vi "Vision Processing Broken.vi"(4 "error in (no error)":errorcluster, 7 "Image Size":T1=enum."320x240") -> ()   [LabVIEW 2015]
doc: "This VI runs in parallel to other tasks. It gets images from the camera, processes them for color or shape and uses commands or globals to affect the behavior of other subsystems."
uses:
  <vilib>/Rock Robotics/WPI/Camera/WPI_CameraImageSize.ctl
  Vision Support Code/Camera Types.ctl
  <vilib>/Rock Robotics/WPI/Camera/WPI_CameraWhite Balance Values.ctl
  <vilib>/Rock Robotics/WPI/Camera/WPI_CameraExposure Values.ctl
  <vilib>/Rock Robotics/WPI/Camera/WPI_CameraFrameRate.ctl
  Framework/Robot Global Data.vi
  Drive/Implementation/Global Drive Variables.vi
  LED Lights/LED Lights Global.vi
  <vilib>/vision/NI_Vision_Development_Module.lvlib
panel:
  out "error out 2":errorcluster
  out "error out":errorcluster
  out "Vision Enabled":bool
  in  "Max Limit %":dbl=0.12 format="%#_13g"
  in  "Min Limit %":dbl=0.12 format="%#_13g"
  in  "Image Size 2":T1=enum."320x240"
  out "ms to process 2":u32
  in  "error in (no error) 2":errorcluster
  out "ms to process":u32
  in  "LED Color":T2={"Hue"={23.67058792990901, 48.923317529462665}, "Sat"={66.78571428571429, 255.0}, "Val"={48.571428571428584, 255.0}} {"Hue" scale=0.0..255.0 scale format="%#_3g"}
  out "Qualified Particles":i32
  in  "Score Threshold":dbl=75.0
  in  "Aspect Fudge Factor":dbl=1.0
  in  "Min Score Threshold":i32=75
  in  "Camera Type":T3=enum."MS HD3000 square"
  in  "Emphasize Limit Tests":bool=TRUE
  out "Masked 2":T4(plugin-control)
  in  "Display Mask":bool=TRUE
  out "Original Image":T4(plugin-control)
  in  "Display Original":bool=TRUE
  out "Sorted Particle Scores":T5(array[cluster]) {"Moment Factor" format="%#_3g"; "Aspect Ratio" format="%#_3g"; "Area to CH" format="%#_3g"; "X" format="%#_3g"; "Y" format="%#_3g"}
  out "Highest Avg Score":dbl
  out "Detected Targets":T6(array[cluster]) {"Normalized Rect"."Numeric 5" format="%#_2g"; "Normalized Rect"."Numeric 3" format="%#_2g"; "Normalized Rect"."Numeric 2" format="%#_2g"; "Normalized Rect"."Numeric" format="%#_2g"}
  out "fps":dbl
  out "Masked":T4(plugin-control)
  # "Density Profile"
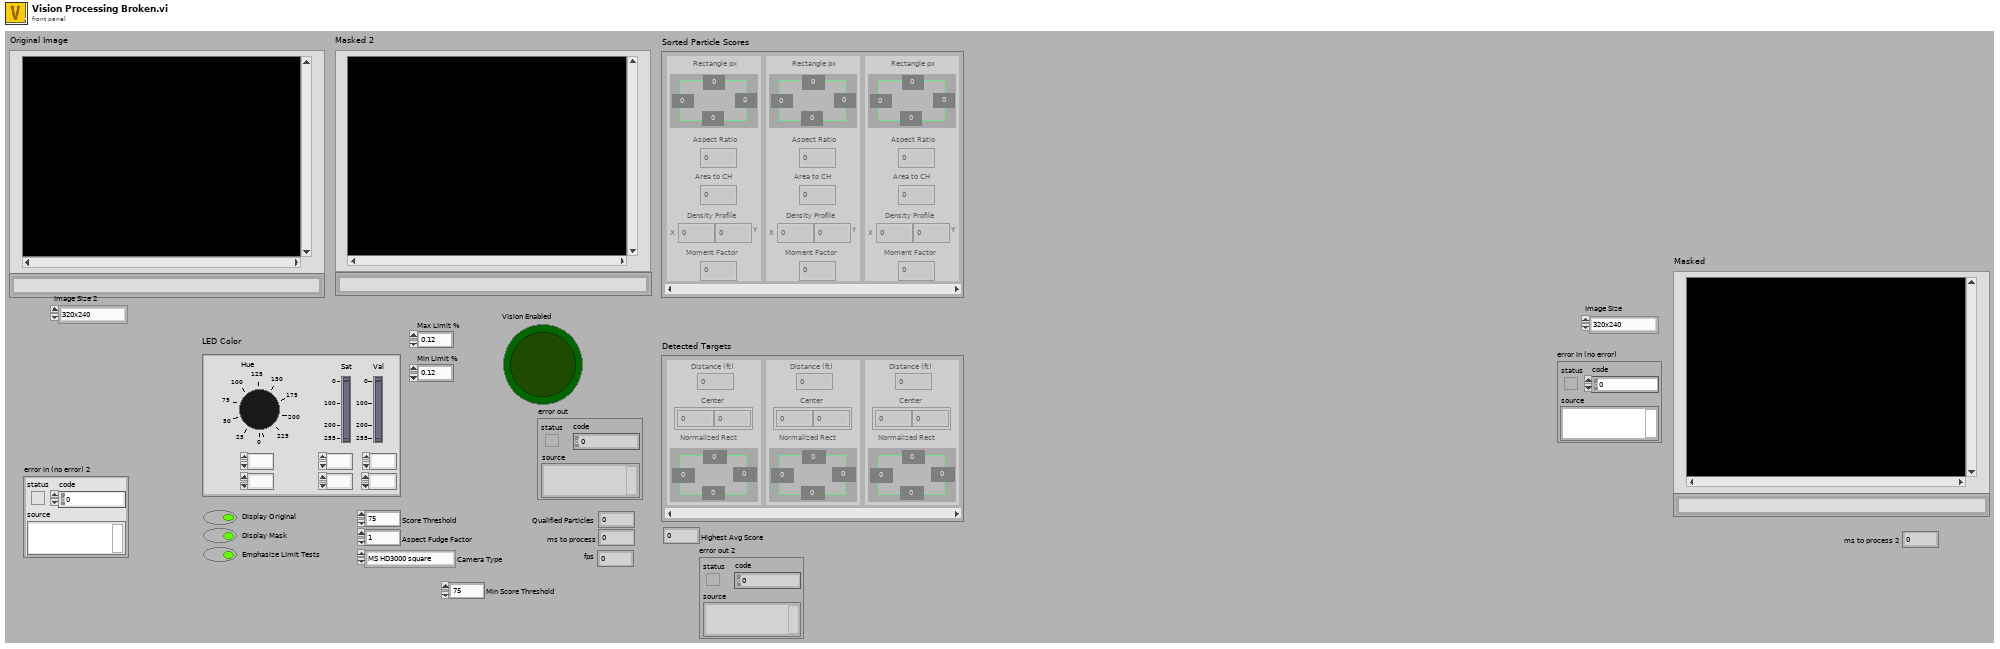
[diagram p1: front panel]
types:
  T1 = typedef "WPI_CameraImageSize.ctl" = enum16{"640x480", "320x240", "160x120", "Custom"}
  T2 = cluster{"Hue":cluster{dbl, dbl}, "Sat":cluster{dbl, dbl}, "Val":cluster{dbl, dbl}}
  T3 = typedef "Camera Types.ctl" = enum16{"206", "1011", "1013", "MS HD3000 square", "MS HD3000 640x480"}
  T4 = typedef "IMAQ Image.ctl" = refnum<image>
  T5 = cluster{"Rectangle px":cluster{"Numeric":dbl, "Numeric 2":dbl, "Numeric 3":dbl, "Numeric 5":dbl}, "Aspect Ratio":dbl, "Area to CH":dbl, "X":dbl, "Y":dbl, "Moment Factor":dbl}[]
  T6 = cluster{"Distance (ft)":dbl, "Center":cluster{dbl, dbl}, "Normalized Rect":cluster{"Numeric":dbl, "Numeric 2":dbl, "Numeric 3":dbl, "Numeric 5":dbl}}[]
  T7 = typedef "WPI_CameraFrameRate.ctl" = u32
  T8 = typedef "WPI_CameraExposure Values.ctl" = enum16{"Auto", "Flicker-free 50 Hz", "Flicker-free 60 Hz", "Hold current", "Custom"}
  T9 = typedef "WPI_CameraWhite Balance Values.ctl" = enum16{"Auto", "Fixed indoor", "Fixed outdoor 1", "Fixed outdoor 2", "Fixed fluorescent 1", "Fixed fluorescent 2", "Hold current", "Custom"}
  T10 = typedef "WPI_CameraDevRef.ctl" = cluster{"Camera Address":string, "CameraStatus":errorcluster}
  T11 = typedef "Image Type" = u32
  T12 = typedef "Particle Parameters" = i32
  T13 = cluster{"Bounding box":cluster{"left":dbl, "top":dbl, "right":dbl, "bottom":dbl}, "Aspect Ratio":dbl, "Area to CH":dbl, "X Mask":dbl, "Y Mask":dbl, "Moment":dbl}[]
  T14 = cluster{"Rectangle":cluster{"Numeric":dbl, "Numeric 2":dbl, "Numeric 3":dbl, "Numeric 5":dbl}, "L":dbl, "Area to CH":dbl, "X":dbl, "Y":dbl, "Moment Factor":dbl}[]
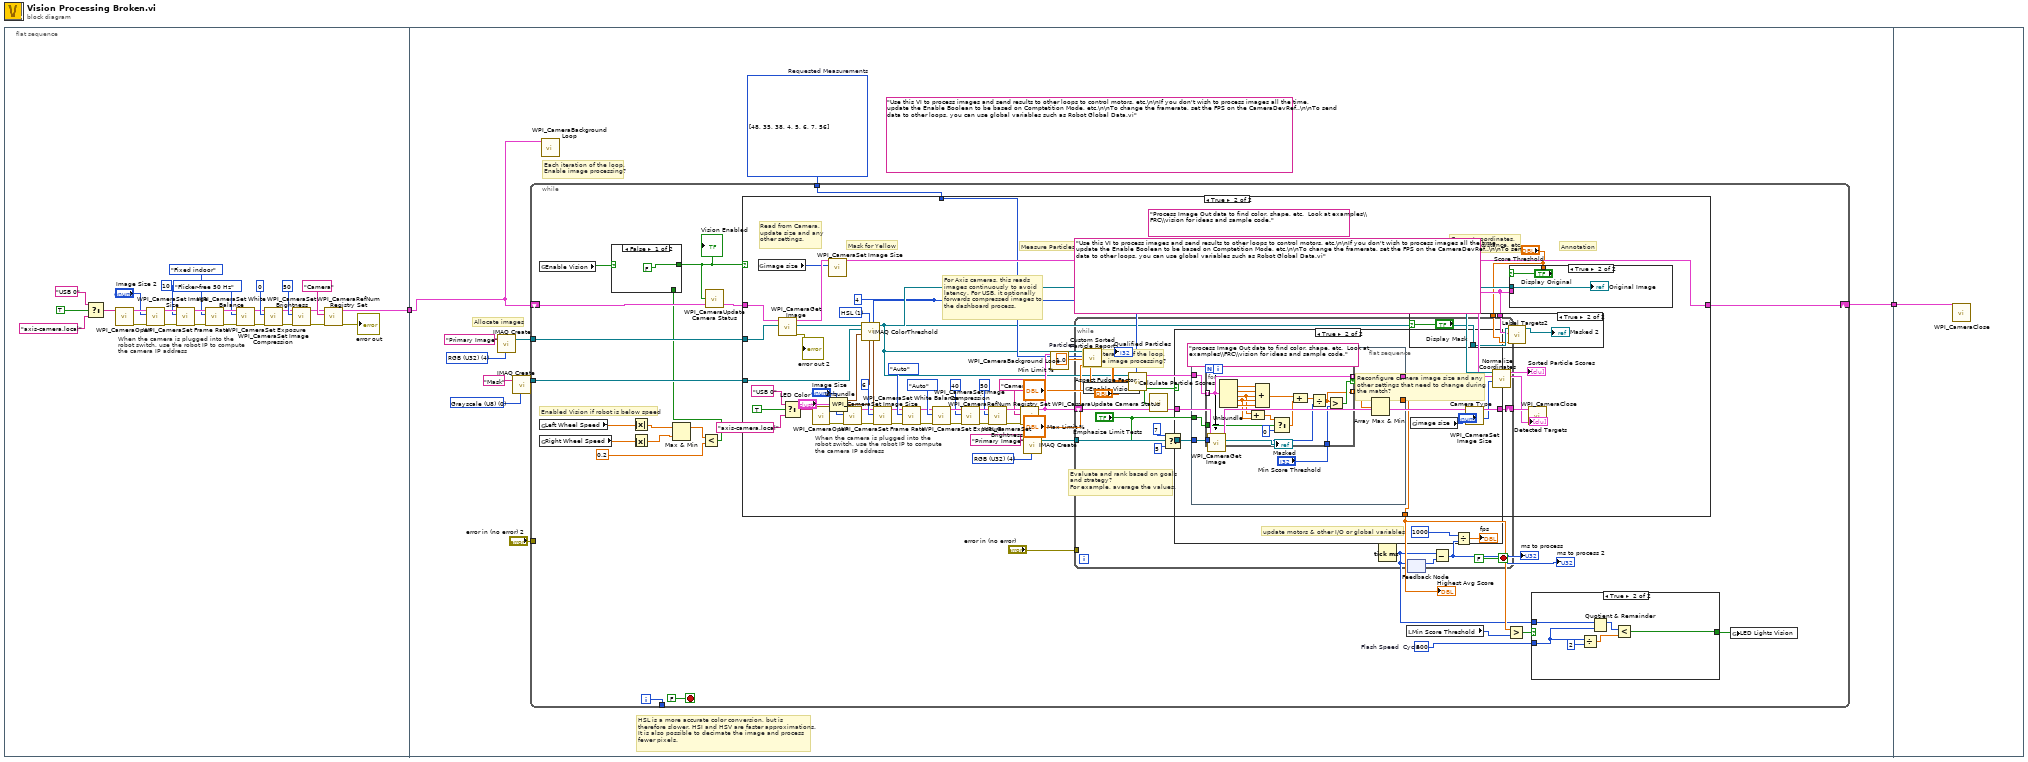
[diagram p0: block diagram]
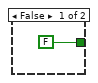
[diagram p2: hidden frame]
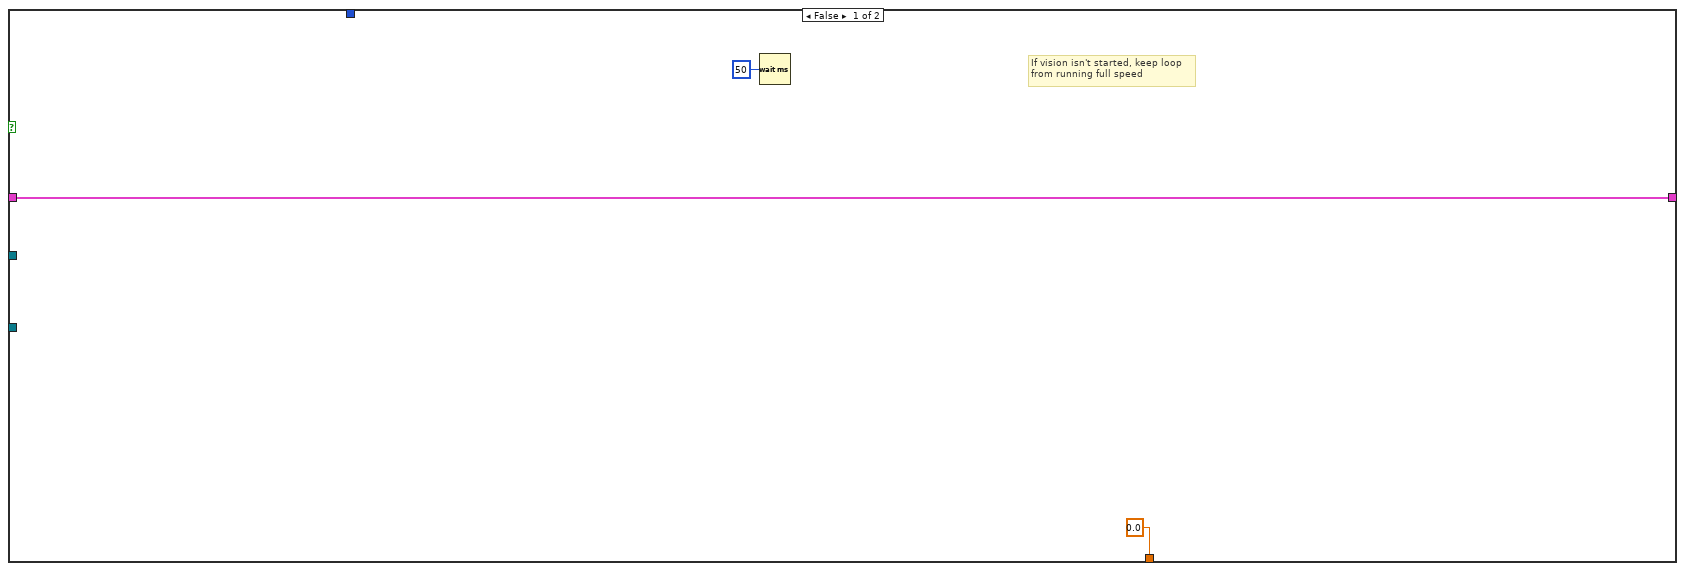
[diagram p4: hidden frame]
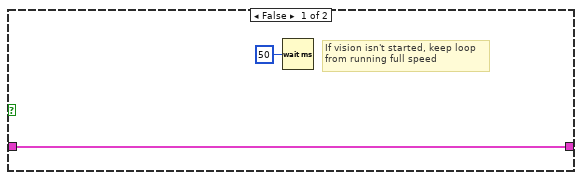
[diagram p7: hidden frame]
diagram:
  n1 = flat-sequence {
    tunnel: [w4] -> w2
    tunnel: w2 -> [w31]
    tunnel: [w30] -> w1
    tunnel: w1 -> [w187]
    frame #0 {
      # "When the camera is plugged into the\nrobot switch, use the robot IP to compute\nthe camera IP address"
      n2 = Select(t="USB 0" ("format string"), s=TRUE ("dot notation? (F)"), f="axis-camera.local" ("format string")) -> (s? t:f=w6:string)
      n3 = call <vilib>:"WPI_CameraOpen.vi"("Camera Address"=w6) -> ("error out"=w20:errorcluster, "CameraDevRef"=w21:T10)  [unwired: 1 in, 8 out]
      n4 = call <vilib>:"WPI_CameraSet Image Size.vi"("error in (no error)"=w20, "Image Size"="Image Size 2", "CameraDevRef"=w21) -> ("error out"=w19:errorcluster, "CameraDevRef Out"=w22:T10)  [unwired: 1 in, 6 out]
      n5 = call <vilib>:"WPI_CameraSet Frame Rate.vi"("error in (no error)"=w19, "Frame Rate (fps)"=T7 10, "CameraDevRef"=w22) -> ("error out"=w18:errorcluster, "CameraDevRef Out"=w24:T10)  [unwired: 7 out]
      n6 = call <vilib>:"WPI_CameraSet White Balance.vi"("error in (no error)"=w18, "White Balance"=WPI_CameraWhite_Balance_Values."Fixed indoor", "CameraDevRef"=w24) -> ("error out"=w17:errorcluster, "CameraDevRef Out"=w23:T10)  [unwired: 1 in, 6 out]
      n7 = call <vilib>:"WPI_CameraSet Exposure.vi"("error in (no error)"=w17, "Exposure"=WPI_CameraExposure_Values."Flicker-free 50 Hz", "CameraDevRef"=w23) -> ("error out"=w16:errorcluster, "CameraDevRef Out"=w26:T10)  [unwired: 1 in, 6 out]
      n8 = call <vilib>:"WPI_CameraSet Image Compression.vi"("error in (no error)"=w16, "Compression"=0, "CameraDevRef"=w26) -> ("error out"=w15:errorcluster, "CameraDevRef Out"=w25:T10)  [unwired: 7 out]
      n9 = call <vilib>:"WPI_CameraSet Brightness.vi"("error in (no error)"=w15, "Brightness"=50, "CameraDevRef"=w25) -> ("error out"=w13:errorcluster, "CameraDevRef Out"=w14:T10)  [unwired: 7 out]
      n10 = call <vilib>:"WPI_CameraRefNum Registry Set.vi"("error in (no error)"=w13, "refnum name"="Camera", "CameraDevRef"=w14) -> ("error out"=→"error out":errorcluster, "CameraDevRef"=w4:T10)  [unwired: 1 in, 6 out]
    }
    frame #1 {
      w68 = T11 4 items=["Grayscale (U8)", "Grayscale (I16)", "Grayscale (SGL)", "Complex (CSG)", "RGB (U32)", "HSL (U32)", "RGB (U64)"] ("Image Type")
      (unwired) "Use this VI to process images and send results to other loops to control motors, etc.\n\nIf you don't wish to process images all the time, update the Enable Boolean to be based on Comptetition Mode, etc.\n\nTo change the framerate, set the FPS on the CameraDevRef..\n\nTo send data to other loops, you can use global variables such as Robot Global Data.vi"
      w66 = T12[] [48, 35, 38, 4, 5, 6, 7, 56] items=["Center of Mass X", "Center of Mass Y", "First Pixel X", "First Pixel Y", "Bounding Rect Left", "Bounding Rect Top", "Bounding Rect Right", "Bounding Rect Bottom", "Max Feret Diameter Start X", "Max Feret Diameter Start Y", "Max Feret Diameter End X", "Max Feret Diameter End Y", "Max Horiz. Segment Length Left", "Max Horiz. Segment Length Right", "Max Horiz. Segment Length Row", "-", "Bounding Rect Width", "Bounding Rect Height", "Bounding Rect Diagonal", "Perimeter", "Convex Hull Perimeter", "Holes' Perimeter", "Max Feret Diameter", "Equivalent Ellipse Major Axis", "Equivalent Ellipse Minor Axis", "Equivalent Ellipse Minor Axis (Feret)", "Equivalent Rect Long Side", "Equivalent Rect Short Side", "Equivalent Rect Diagonal", "Equivalent Rect Short Side (Feret)", "Average Horiz. Segment Length", "Average Vert. Segment Length", "Hydraulic Radius", "Waddel Disk Diameter", "-", "Area", "Holes' Area", "Particle & Holes' Area", "Convex Hull Area", "Image Area", "-", "Number of Holes", "Number of Horiz. Segments", "Number of Vert. Segments", "-", "Orientation", "Max Feret Diameter Orientation", "-", "% Area/Image Area", "% Area/(Particle & Holes' Area)", "Ratio of Equivalent Ellipse Axes", "Ratio of Equivalent Rect Sides", "-", "Elongation Factor", "Compactness Factor", "Heywood Circularity Factor", "Type Factor", "-", "Sum X", "Sum Y", "Sum XX", "Sum XY", "Sum YY", "Sum XXX", "Sum XXY", "Sum XYY", "Sum YYY", "-", "Moment of Inertia XX", "Moment of Inertia XY", "Moment of Inertia YY", "Moment of Inertia XXX", "Moment of Inertia XXY", "Moment of Inertia XYY", "Moment of Inertia YYY", "Norm. Moment of Inertia XX", "Norm. Moment of Inertia XY", "Norm. Moment of Inertia YY", "Norm. Moment of Inertia XXX", "Norm. Moment of Inertia XXY", "Norm. Moment of Inertia XYY", "Norm. Moment of Inertia YYY", "Hu Moment 1", "Hu Moment 2", "Hu Moment 3", "Hu Moment 4", "Hu Moment 5", "Hu Moment 6", "Hu Moment 7"]  # Requested Measurements
      w63 = T11 0 items=["Grayscale (U8)", "Grayscale (I16)", "Grayscale (SGL)", "Complex (CSG)", "RGB (U32)", "HSL (U32)", "RGB (U64)", "Grayscale (U16)"] ("Image Type")
      (unwired) "Use this VI to process images and send results to other loops to control motors, etc.\n\nIf you don't wish to process images all the time, update the Enable Boolean to be based on Comptetition Mode, etc.\n\nTo change the framerate, set the FPS on the CameraDevRef..\n\nTo send data to other loops, you can use global variables such as Robot Global Data.vi"
      w32 = T11 4 items=["Grayscale (U8)", "Grayscale (I16)", "Grayscale (SGL)", "Complex (CSG)", "RGB (U32)", "HSL (U32)", "RGB (U64)"] ("Image Type")
      # "Each iteration of the loop,\nEnable image processing?"
      # "HSL is a more accurate color conversion, but is\ntherefore slower. HSI and HSV are faster approximations.\nIt is also possible to decimate the image and process\nfewer pixels."
      # "Allocate images"
      # "When the camera is plugged into the\nrobot switch, use the robot IP to compute\nthe camera IP address"
      # "For Axis cameras, this reads\nimages continuously to avoid\nlatency. For USB, it optionally\nforwards compressed images to\nthe dashboard process."
      n11 = call "IMAQ Create"("Image Name"="Primary Image", "Image Type"=w68) -> ("New Image"=w70:T4)  [unwired: 2 in, 2 out]
      n12 = call "IMAQ Create"("Image Name"="Mask", "Image Type"=w63) -> ("New Image"=w65:T4)  [unwired: 2 in, 2 out]
      n13 = while {
        tunnel: w70 -> [w93]
        tunnel: w65 -> [w96]
        tunnel: w66 -> [w95]
        tunnel: "error in (no error) 2" -> [_]
        tunnel: [w92] -> _
        shift-right: [w90] -> w30
        shift-left: w31 -> [w86]
        i -> [w92]
        stop <- FALSE stop-if-true
        w73 = 500  # Flash Speed  Cycle
        # "Enabled Vision if robot is below speed"
        n14 = global read "Robot Global Data.vi" "Enable Vision"() -> (w83:bool)
        n15 = global read "Global Drive Variables.vi" "Left Wheel Speed"() -> (w79:dbl)
        n16 = global read "Global Drive Variables.vi" "Right Wheel Speed"() -> (w78:dbl)
        n17 = Absolute Value(x=w79) -> (abs(x)=w80:dbl)
        n18 = Absolute Value(x=w78) -> (abs(x)=w77:dbl)
        n19 = Max & Min(x=w80, y=w77) -> (max(x,y)=w85:dbl)  [unwired: 1 out]
        n20 = Less?(x=w85, y=0.2) -> (x < y?=w81:bool)
        n21 = case shown="False" w83 {
          tunnel: [FALSE w106] -> w82
          tunnel: w81 -> [_ w106]
          frame False {
          }
          frame True {
          }
        }
        "Vision Enabled" <- w82
        n22 = call <vilib>:"WPI_CameraUpdate Camera Status.vi"("CameraDevRef In"=w86, "Enable Vision"=w82) -> ("CameraDevRef Out"=w91:T10)  [unwired: 3 in]
        n23 = case shown="True" w82 {
          tunnel: w96 -> [_ w144]
          tunnel: w95 -> [_ w116]
          tunnel: w91 -> [w108 w139]
          tunnel: w93 -> [_ w138]
          tunnel: [w108 w136] -> w90
          tunnel: [0.0 w111] -> w75
          frame False {
            # "If vision isn't started, keep loop\nfrom running full speed"
            n24 = Wait (ms)(milliseconds to wait=u32 50) -> ()  [unwired: 1 out]
          }
          frame True {
            w124 = 4 ("Replace Value")
            w133 = u16 1 items=["RGB", "HSL", "HSV", "HSI"] ("Color Mode")
            (unwired) "Process Image Out data to find color, shape, etc.  Look at examples\\FRC\\vision for ideas and sample code."
            w114 = 1.0  # Particles
            # "Evaluate and rank based on goals\nand strategy?\nFor example, average the values."
            # "Read from Camera,\nupdate size and any\nother settings."
            # "Measure Particles"
            # "Convert coordinates,\ncalculate distance, etc."
            # "Annotation"
            # "Score Particles"
            # "Mask for Yellow"
            n25 = global read "Robot Global Data.vi" "image size"() -> (w121:T1)
            n26 = call <vilib>:"WPI_CameraGet Image.vi"("Image"=w138, "CameraDevRef"=w139) -> ("error out"=→"error out 2":errorcluster, "Image Out"=w125:T4, "CameraDevRef Out"=w137:T10)  [unwired: 7 in]
            n27 = call <vilib>:"WPI_CameraSet Image Size.vi"("Image Size"=w121, "CameraDevRef"=w137) -> ("CameraDevRef Out"=w136:T10)  [unwired: 2 in, 7 out]
            n28 = Unbundle("LED Color") -> ("Hue"=w143:cluster{dbl, dbl}, "Sat"=w142:cluster{dbl, dbl}, "Val"=w141:cluster{dbl, dbl})
            n29 = call "IMAQ ColorThreshold"("Blue or Luma or Val or Inten Range"=w141, "Replace Value"=w124, "Green or Sat Range"=w142, "Color Mode"=w133, "Red or Hue Range"=w143, "Image Dst"=w144, "Image Src"=w125) -> ("Image Dst Out"=w112:T4)  [unwired: 3 in, 1 out]
            n30 = call "Custom Sorted Particle Report.vi"("Min Area Size %"="Min Limit %", "Max Area Size %"="Max Limit %", "Particle Count Limit"=w114, "Pixel Measurements"=w116, "Image in"=w112) -> ("Particles"=→"Qualified Particles":i32, "Sorted Data"=w117:dbl[][])  [unwired: 5 in]
            n31 = call "Calculate Particle Scores.vi"("Pixel Value"=w124, "Aspect Fudge Factor"="Aspect Fudge Factor", "Sorted Data"=w117, "Image in"=w112) -> ("Scores"=w131:T13)  [unwired: 7 in]
            n32 = Select(t=7, s="Emphasize Limit Tests", f=5) -> (s? t:f=w128:i32)
            n33 = flat-sequence {
              tunnel: w131 -> [w155]
              tunnel: w128 -> [w153]
              tunnel: [w156] -> w111
              tunnel: [w150] -> w120
              tunnel: "Emphasize Limit Tests" -> [w154]
              frame #0 {
                n34 = for {
                  tunnel: w155 -> [w170] mode=indexing
                  tunnel: [w170] -> w150 mode=indexing if=w169
                  tunnel: [w168] -> w151 mode=indexing
                  tunnel: w153 -> [w167]
                  tunnel: "Min Score Threshold" -> [w166]
                  tunnel: w154 -> [w159]
                  n35 = Unbundle(w170) -> ("Aspect Ratio"=w172:dbl, "Area to CH"=w171:dbl, "X Mask"=w161:dbl, "Y Mask"=w162:dbl, "Moment"=w163:dbl)  [unwired: 1 out]
                  n36 = Compound Arithmetic op=ADD(w161, w162) -> (w160:dbl)
                  n37 = Compound Arithmetic op=ADD(w172, w171, w161, w162, w163) -> (w165:dbl)
                  n38 = Select(t=w160, s=w159, f=0) -> (s? t:f=w158:dbl)
                  n39 = Compound Arithmetic op=ADD(w165, w158) -> (w164:dbl)
                  n40 = Divide(x=w164, y=w167) -> (x/y=w168:dbl)
                  n41 = Greater?(x=w168, y=w166) -> (0:w169:bool)
                }
                n42 = Array Max & Min(array=w151) -> (max value=w156:dbl)  [unwired: 3 out]
              }
            }
            n43 = case shown="True" "Display Mask" {
              tunnel: w112 -> [_ w149]
              tunnel: w120 -> [_ w147]
              tunnel: "Score Threshold" -> [_ w146]
              frame False {
              }
              frame True {
                n44 = call "Label Targets2.vi"("Score Threshold"=w146, "Targets"=w147, "Image in"=w149) -> ("Image out"=→"Masked 2":T4)  [unwired: 8 in]
              }
            }
            n45 = call "Normalize Coordinates.vi"("Camera Type"="Camera Type", "Targets"=w120, "Image in"=w125) -> ("Found Targets"=→"Detected Targets":T6, "Sorted Scores"=→"Sorted Particle Scores":T14)  [unwired: 7 in]
            n46 = case shown="True" "Display Original" {
              tunnel: w125 -> [_ w145]
              tunnel: w120 -> [_ _]
              tunnel: "Score Threshold" -> [_ _]
              frame False {
              }
              frame True {
                "Original Image" <- w145
              }
            }
          }
        }
        "Highest Avg Score" <- w75
        n47 = Tick Count (ms)() -> (millisecond timer value=w74:u32)
        n48 = local read "Min Score Threshold"() -> (w71:i32)
        n49 = feedback-in #1(w74) -> ()
        n50 = feedback #1() -> (w94:u32)  [unwired: 1 in]
        n51 = Subtract(x=w74, y=w94) -> (x-y=w87:u32)
        "ms to process" <- w87
        "ms to process 2" <- w87
        n52 = Divide(x=1000 ("Brightness"), y=w87) -> (x/y=→"fps":dbl)
        n53 = Greater?(x=w75, y=w71) -> (0:w76:bool)
        n54 = case shown="True" w76 {
          tunnel: w74 -> [_ w103]
          tunnel: [FALSE w102] -> w72
          tunnel: w73 -> [_ w100]
          frame False {
          }
          frame True {
            n55 = Divide(x=w100, y=2) -> (x/y=w101:dbl)
            n56 = Quotient & Remainder(x=w103, y=w100) -> (x-y*floor(x/y)=w104:u32)  [unwired: 1 out]
            n57 = Less?(x=w104, y=w101) -> (x < y?=w102:bool)
          }
        }
        n58 = global write "LED Lights Global.vi" "LED Lights Vision"(w72) -> ()
      }
      n59 = call <vilib>:"WPI_CameraBackground Loop.vi"("CameraDevRef"=w31) -> ()  [unwired: 11 in]
      n60 = Select(t="USB 0" ("format string"), s=TRUE ("dot notation? (F)"), f="axis-camera.local" ("format string")) -> (s? t:f=w61:string)
      n61 = call <vilib>:"WPI_CameraOpen.vi"("Camera Address"=w61) -> ("error out"=w44:errorcluster, "CameraDevRef"=w43:T10)  [unwired: 1 in, 8 out]
      n62 = call <vilib>:"WPI_CameraSet Image Size.vi"("error in (no error)"=w44, "Image Size"="Image Size", "CameraDevRef"=w43) -> ("error out"=w45:errorcluster, "CameraDevRef Out"=w42:T10)  [unwired: 1 in, 6 out]
      n63 = call <vilib>:"WPI_CameraSet Frame Rate.vi"("error in (no error)"=w45, "Frame Rate (fps)"=T7 6, "CameraDevRef"=w42) -> ("error out"=w46:errorcluster, "CameraDevRef Out"=w40:T10)  [unwired: 7 out]
      n64 = call <vilib>:"WPI_CameraSet White Balance.vi"("error in (no error)"=w46, "White Balance"=WPI_CameraWhite_Balance_Values."Auto", "CameraDevRef"=w40) -> ("error out"=w47:errorcluster, "CameraDevRef Out"=w41:T10)  [unwired: 1 in, 6 out]
      n65 = call <vilib>:"WPI_CameraSet Exposure.vi"("error in (no error)"=w47, "Exposure"=WPI_CameraExposure_Values."Auto", "CameraDevRef"=w41) -> ("error out"=w48:errorcluster, "CameraDevRef Out"=w38:T10)  [unwired: 1 in, 6 out]
      n66 = call <vilib>:"WPI_CameraSet Image Compression.vi"("error in (no error)"=w48, "Compression"=40, "CameraDevRef"=w38) -> ("error out"=w49:errorcluster, "CameraDevRef Out"=w39:T10)  [unwired: 7 out]
      n67 = call <vilib>:"WPI_CameraSet Brightness.vi"("error in (no error)"=w49, "Brightness"=50, "CameraDevRef"=w39) -> ("error out"=w51:errorcluster, "CameraDevRef Out"=w50:T10)  [unwired: 7 out]
      n68 = call <vilib>:"WPI_CameraRefNum Registry Set.vi"("error in (no error)"=w51, "refnum name"="Camera", "CameraDevRef"=w50) -> ("CameraDevRef"=w55:T10)  [unwired: 1 in, 7 out]
      n69 = call "IMAQ Create"("Image Name"="Primary Image", "Image Type"=w32) -> ("New Image"=w34:T4)  [unwired: 2 in, 2 out]
      n70 = call <vilib>:"WPI_CameraBackground Loop.vi"("CameraDevRef"=w55) -> ()  [unwired: 11 in]
      n71 = while {
        shift-right: [w177] -> w57
        shift-left: w55 -> [w175]
        tunnel: w34 -> [w176]
        tunnel: "error in (no error)" -> [_]
        stop <- FALSE stop-if-true
        # "Each iteration of the loop,\nEnable image processing?"
        n72 = global read "Robot Global Data.vi" "Enable Vision"() -> (w173:bool)
        n73 = call <vilib>:"WPI_CameraUpdate Camera Status.vi"("CameraDevRef In"=w175, "Enable Vision"=w173) -> ("CameraDevRef Out"=w174:T10)  [unwired: 3 in]
        n74 = case shown="True" w173 {
          tunnel: w176 -> [_ w185]
          tunnel: [w180 w186] -> w177
          tunnel: w174 -> [w180 w183]
          frame False {
            # "If vision isn't started, keep loop\nfrom running full speed"
            n75 = Wait (ms)(milliseconds to wait=u32 50) -> ()  [unwired: 1 out]
          }
          frame True {
            (unwired) "process Image Out data to find color, shape, etc.  Look at examples\\FRC\\vision for ideas and sample code."
            # "update motors & other I/O or global variables"
            # "Reconfigure camera image size and any\nother settings that need to change during\nthe match?"
            n76 = call <vilib>:"WPI_CameraGet Image.vi"("Image"=w185, "CameraDevRef"=w183) -> ("Image Out"=→"Masked":T4, "CameraDevRef Out"=w182:T10)  [unwired: 1 in, 7 out]
            n77 = global read "Robot Global Data.vi" "image size"() -> (w184:T1)
            n78 = call <vilib>:"WPI_CameraSet Image Size.vi"("Image Size"=w184, "CameraDevRef"=w182) -> ("CameraDevRef Out"=w186:T10)  [unwired: 2 in, 7 out]
          }
        }
      }
      n79 = call <vilib>:"WPI_CameraClose.vi"("CameraDevRef"=w57) -> ()  [unwired: 1 in, 10 out]
    }
    frame #2 {
      n80 = call <vilib>:"WPI_CameraClose.vi"("CameraDevRef"=w187) -> ()  [unwired: 1 in, 10 out]
    }
  }
